vi "datagen.vi"() -> ()   [LabVIEW 2020]
uses:
  <vilib>/Graiphic/HAIBAL Deep learning/Source/Layer/Dense/_Controls/dense_param.ctl
  <vilib>/Graiphic/HAIBAL Deep learning/Source/_Controls/activation_enum.ctl
  <vilib>/Graiphic/HAIBAL Deep learning/Source/_Controls/optimizer_param.ctl
  <vilib>/Graiphic/HAIBAL Deep learning/Source/_Controls/optimizer_enum.ctl
  <vilib>/Graiphic/HAIBAL Deep learning/Source/Init/_Controls/Init_Enum.ctl
  <vilib>/Graiphic/HAIBAL Deep learning/Source/Model/Controls/frw_training_mode.ctl
  <vilib>/Graiphic/HAIBAL Deep learning/Source/Layer/Input/_Methods/add_to_graph.vi
  <vilib>/Graiphic/HAIBAL Deep learning/Source/Layer/Dense/_Methods/add_to_graph.vi
  <vilib>/Graiphic/HAIBAL Deep learning/Source/Model/_Methods/mono_input_2d.vi
  <vilib>/Graiphic/HAIBAL Deep learning/Source/Model/_Methods/mono_y_true_2d.vi
  <vilib>/Graiphic/HAIBAL Deep learning/Source/Model/_Methods/backward.vi
  <vilib>/Graiphic/HAIBAL Deep learning/Source/Model/_Methods/get_2d_output_frw.vi
  <vilib>/Graiphic/HAIBAL Deep learning/Source/Layer/Dense/Dense.lvclass
  <vilib>/Graiphic/HAIBAL Deep learning/Source/Model/Model.lvclass
  <vilib>/Graiphic/HAIBAL Deep learning/Source/Layer/Input/Input.lvclass
panel:
  out "Waveform Chart":sgl(graph)
  out "Epoch":i32
  out "Graph Display":cluster{"X":sgl, "Y_True":sgl, "Y_Pred":sgl}[](graph)
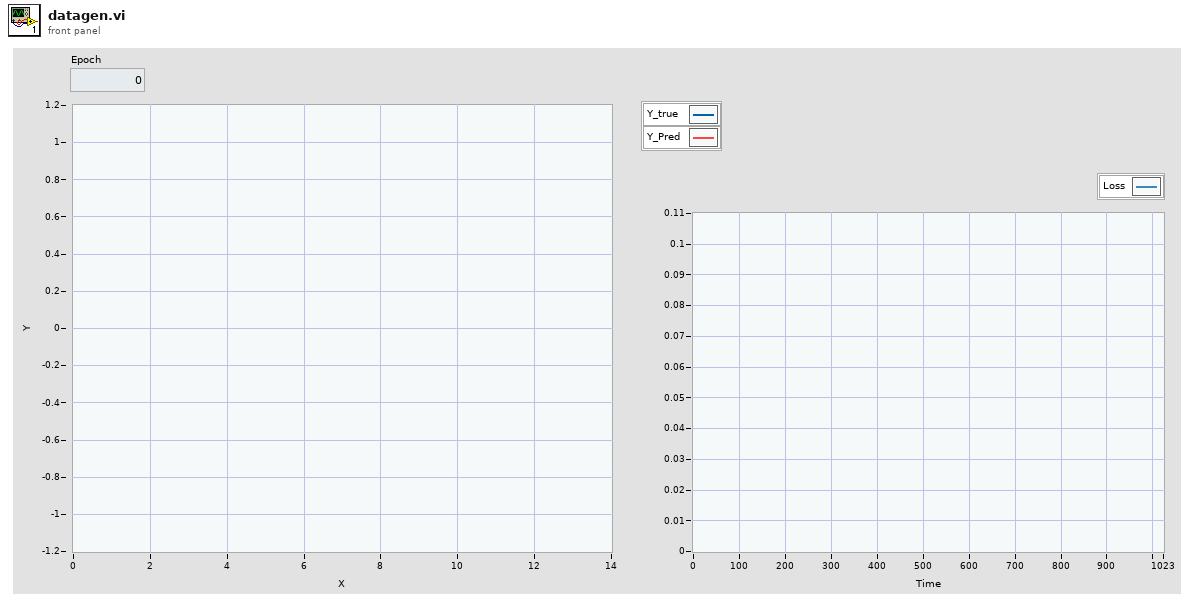
[diagram p1: front panel]
types:
  T1 = typedef "Dense.lvclass/dense_param.ctl" = cluster{"units":i32, "activation":T2, "use_bias?":bool, "optimizer":T3, "weight_initializer":T5, "bias_initializer":T5, "training?":bool, "store?":bool, "update?":bool, "lda_coeff":dbl}
  T2 = typedef "activation_enum.ctl" = enum16{"elu", "exponential", "gelu", "hard_sigmoid", "leaky_relu", "linear", "relu", "selu", "sigmoid", "softmax", "softplus", "softsign", "swish", "tanh", "thresholdedrelu"}
  T3 = typedef "optimizer_param.ctl" = cluster{"algorithm":T4, "learning_rate":sgl, "beta_1":sgl, "beta_2":sgl}
  T4 = typedef "optimizer_enum.ctl" = enum16{"adadelta", "adagrad", "adam", "adamax", "inertia", "nadam", "nesterov", "rmsprop", "sgd"}
  T5 = typedef "Init_Enum.ctl" = enum16{"Constant", "GlorotNormal", "GlorotUniform", "HeNormal", "HeUniform", "Identity", "LeCunNormal", "LeCunUniform", "Ones", "Orthogonal", "RandomNormal", "RandomUniform", "TruncatedNormal", "VarianceScaling", "Zeros"}
  T6 = typedef "frw_training_mode.ctl" = enum16{"Nothing", "Training", "Predict"}
  T7 = typedef "loss_data_cluster.ctl" = cluster{"loss":sgl, "loss_derivate":T8[]}
  T8 = typedef "backward_output_cluster.ctl" = cluster{"name":string, "index":i32, "dimension":T9, "shape":i32[], "data":variant}
  T9 = typedef "loss_der_dimension_enum.ctl" = enum16{"2D Loss Derivate", "3D Loss Derivate", "4D Loss Derivate", "5D Loss Derivate", "6D Loss Derivate"}
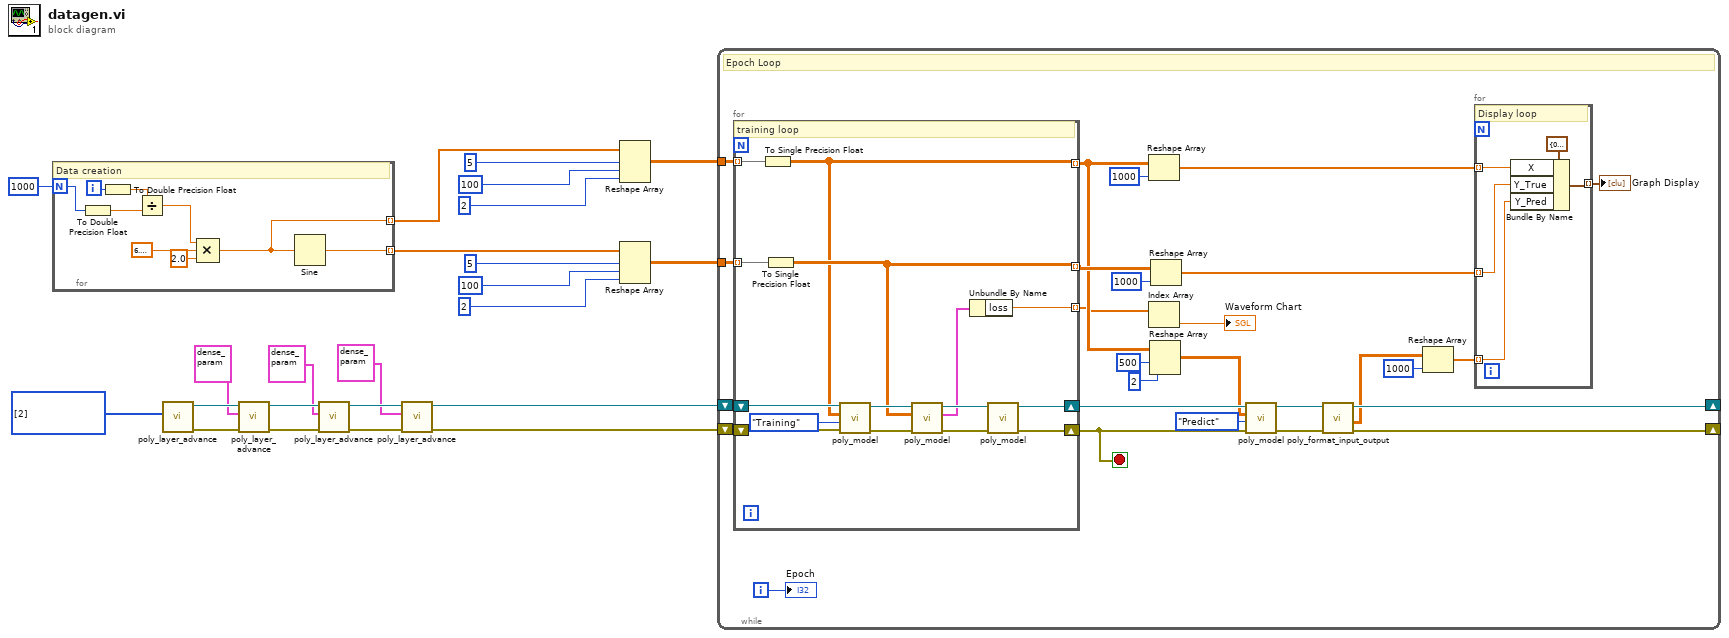
[diagram p0: block diagram]
diagram:
  n1 = for {
    N: 1000 -> [w29]
    tunnel: [w24] -> w5 mode=indexing
    tunnel: [w25] -> w12 mode=indexing
    i -> [w30]
    # "Data creation"
    n2 = To Double Precision Float(number=w29) -> (double precision float=w28:dbl)
    n3 = To Double Precision Float(number=w30) -> (double precision float=w27:dbl)
    n4 = Divide(x=w27, y=w28) -> (x/y=w26:dbl)
    n5 = Compound Arithmetic op=MULTIPLY(w26, 6.283185307179586, 2.0 ("value")) -> (w25:dbl)
    n6 = Sine(x=w25) -> (sin(x)=w24:dbl)
  }
  n7 = call-poly <vilib>:"poly_layer_advance.vi"("input_shape"=i32[] [2]) -> ("error out"=w17:errorcluster, "Graph out"=w18:refnum<class "Model.lvclass">)  [unwired: 9 in]
  n8 = call-poly <vilib>:"poly_layer_advance.vi"("error in"=w17, "parameters"=T1 {"units"=150, "activation"=enum."swish", "use_bias?"=TRUE, "optimizer"={"algorithm"=enum."adam", "learning_rate"=0.001, "beta_1"=0.9, "beta_2"=0.999}, "weight_initializer"=enum."GlorotUniform", "bias_initializer"=enum."Zeros", "training?"=TRUE, "store?"=FALSE, "update?"=TRUE, "lda_coeff"=1.0}, "Graph in"=w18) -> ("error out"=w21:errorcluster, "Graph out"=w22:refnum<class "Model.lvclass">)  [unwired: 7 in]
  n9 = call-poly <vilib>:"poly_layer_advance.vi"("error in"=w21, "parameters"=T1 {"units"=150, "activation"=enum."relu", "use_bias?"=TRUE, "optimizer"={"algorithm"=enum."adam", "learning_rate"=0.001, "beta_1"=0.9, "beta_2"=0.999}, "weight_initializer"=enum."GlorotUniform", "bias_initializer"=enum."Zeros", "training?"=TRUE, "store?"=FALSE, "update?"=TRUE, "lda_coeff"=1.0}, "Graph in"=w22) -> ("error out"=w19:errorcluster, "Graph out"=w20:refnum<class "Model.lvclass">)  [unwired: 7 in]
  n10 = call-poly <vilib>:"poly_layer_advance.vi"("error in"=w19, "parameters"=T1 {"units"=2, "activation"=enum."linear", "use_bias?"=TRUE, "optimizer"={"algorithm"=enum."adam", "learning_rate"=0.001, "beta_1"=0.9, "beta_2"=0.999}, "weight_initializer"=enum."GlorotUniform", "bias_initializer"=enum."Zeros", "training?"=TRUE, "store?"=FALSE, "update?"=TRUE, "lda_coeff"=1.0}, "Graph in"=w20) -> ("error out"=w1:errorcluster, "Graph out"=w2:refnum<class "Model.lvclass">)  [unwired: 7 in]
  n11 = Reshape Array(w12, 5 ("dimension size"), 100 ("dimension size"), 2 ("dimension size")) -> (w4:dbl[][][])
  n12 = Reshape Array(w5, 5 ("dimension size"), 100 ("dimension size"), 2 ("dimension size")) -> (w3:dbl[][][])
  n13 = while {
    tunnel: w4 -> [w58]
    tunnel: w3 -> [w57]
    shift-right: [w48] -> _
    shift-left: w2 -> [w56]
    shift-right: [w51] -> _
    shift-left: w1 -> [w55]
    i -> [w59]
    stop <- w54 stop-if-true
    # "Epoch Loop"
    n14 = for {
      tunnel: w58 -> [w76] mode=indexing
      tunnel: w57 -> [w73] mode=indexing
      shift-right: [w70] -> w53
      shift-left: w56 -> [w79]
      shift-right: [w69] -> w54
      shift-left: w55 -> [w78]
      tunnel: [w68] -> w45 mode=indexing
      tunnel: [w67] -> w42 mode=indexing
      tunnel: [w65] -> w34 mode=indexing
      # "training loop"
      n15 = To Single Precision Float(number=w76) -> (single precision float=w67:sgl[][])
      n16 = To Single Precision Float(number=w73) -> (single precision float=w68:sgl[][])
      n17 = call-poly <vilib>:"poly_model.vi"("error in"=w78, "train_mode"=frw_training_mode."Training", "data in"=w67, "Model in"=w79) -> ("error out"=w74:errorcluster, "Model out"=w75:refnum<class "Model.lvclass">)  [unwired: 4 in, 2 out]
      n18 = call-poly <vilib>:"poly_model.vi"("error in"=w74, "y_true_data"=w68, "Model in"=w75) -> ("error out"=w71:errorcluster, "loss_data"=w66:T7, "Model out"=w72:refnum<class "Model.lvclass">)  [unwired: 5 in, 1 out]
      n19 = Unbundle By Name(w66) -> ("loss"=w65:sgl)
      n20 = call-poly <vilib>:"poly_model.vi"("error in"=w71, "Model in"=w72) -> ("error out"=w69:errorcluster, "Model out"=w70:refnum<class "Model.lvclass">)  [unwired: 6 in, 2 out]
    }
    n21 = Reshape Array(w42, 1000 ("dimension size")) -> (w38:sgl[])
    n22 = Index Array(array=w34) -> (element=→"Waveform Chart":sgl)  [unwired: 1 in]
    n23 = Reshape Array(w42, 500 ("dimension size"), 2 ("dimension size")) -> (w43:sgl[][])
    n24 = Reshape Array(w45, 1000 ("dimension size")) -> (w37:sgl[])
    n25 = call-poly <vilib>:"poly_model.vi"("error in"=w54, "train_mode"=frw_training_mode."Predict", "data in"=w43, "Model in"=w53) -> ("error out"=w50:errorcluster, "Model out"=w49:refnum<class "Model.lvclass">)  [unwired: 4 in, 2 out]
    n26 = call-poly <vilib>:"poly_format_input_output.vi"("error in"=w50, "Model in"=w49) -> ("error out"=w51:errorcluster, "output_2d"=w39:sgl[][], "Model out"=w48:refnum<class "Model.lvclass">)  [unwired: 6 in, 1 out]
    n27 = Reshape Array(w39, 1000 ("dimension size")) -> (w36:sgl[])
    n28 = for {
      tunnel: w38 -> [w63] mode=indexing
      tunnel: w37 -> [w62] mode=indexing
      tunnel: w36 -> [w61] mode=indexing
      tunnel: [w60] -> w35 mode=indexing
      # "Display loop"
      n29 = Bundle By Name(cluster=cluster{"X":sgl, "Y_True":sgl, "Y_Pred":sgl} {"X"=0.0, "Y_True"=0.0, "Y_Pred"=0.0}, "X"=w63, "Y_True"=w62, "Y_Pred"=w61) -> (w60:cluster{"X":sgl, "Y_True":sgl, "Y_Pred":sgl})
    }
    "Graph Display" <- w35
    "Epoch" <- w59
  }
